vi "Generate timestamp.vi"(7 "New file":bool, 9 "Time since acquisition start (us)":i32=1, 11 "Timestamp at trial start":timestamp) -> (1 "Date-time string (micro-second precision)":string, 3 "Timestamp at trial start":timestamp)   [LabVIEW 2020]
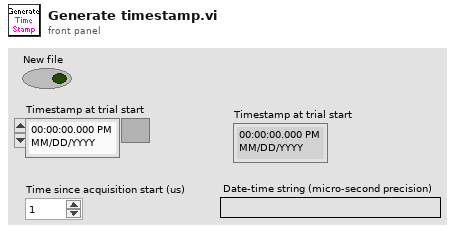
[diagram p1: front panel]
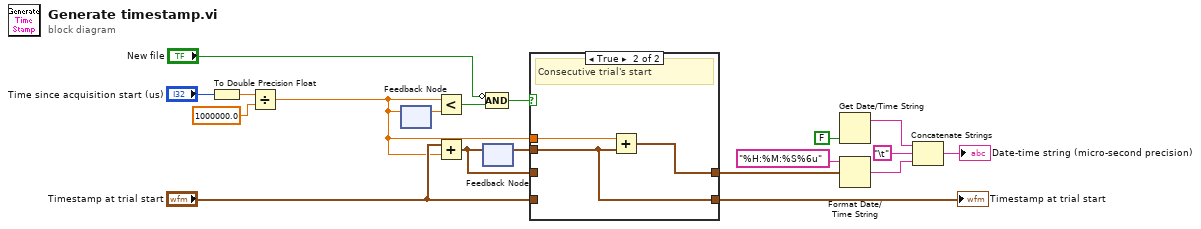
[diagram p0: block diagram]
diagram:
  n1 = To Double Precision Float(number="Time since acquisition start (us)") -> (double precision float=w11:dbl)
  n2 = Divide(x=w11, y=1000000.0) -> (x/y=w3:dbl)
  n3 = feedback #1() -> (w10:dbl)  [unwired: 1 in]
  n4 = feedback-in #1(w3) -> ()
  n5 = Less?(x=w3, y=w10) -> (x < y?=w7:bool)
  n6 = Add(x="Timestamp at trial start", y=w3) -> (x+y=w1:timestamp)
  n7 = feedback #2() -> (w4:timestamp)  [unwired: 1 in]
  n8 = feedback-in #2(w1) -> ()
  n9 = Compound Arithmetic op=AND(invert "New file", w7) -> (w6:bool)
  n10 = case shown="True" w6 {
    tunnel: [w21 w24] -> w9
    tunnel: w4 -> [_ w24]
    tunnel: "Timestamp at trial start" -> [w21 _]
    tunnel: w3 -> [_ w23]
    tunnel: [w20 w22] -> w2
    tunnel: w1 -> [w20 _]
    frame False {
    }
    frame True {
      # "Consecutive trial's start"
      n11 = Add(x=w23, y=w24) -> (x+y=w22:timestamp)
    }
  }
  "Timestamp at trial start" <- w9
  n12 = Get Date/Time String(want seconds? (F)=FALSE) -> (date string=w15:string)  [unwired: 2 in, 1 out]
  n13 = Format Date/Time String(time format string (%c)="%H:%M:%S%6u", seconds (now)=w2) -> (date/time string=w14:string)  [unwired: 1 in]
  n14 = Concatenate Strings(w15, "\t" ("string"), w14) -> (→"Date-time string (micro-second precision)":string)
